vi "FTW-Container-Remove.vi"(0 "Container":refnum<class "FTW-Container.lvclass">, 5 "Value":variant, 11 "error in":errorcluster) -> (4 "Container out":refnum<class "FTW-Container.lvclass">, 6 "Removed?":bool, 8 "Value Removed":variant, 15 "error out":errorcluster)   [LabVIEW 2013, in "FTW-Container.lvclass"]
uses:
  FTW-Container.lvclass
panel:
  # "Inputs"
  # "Outputs"
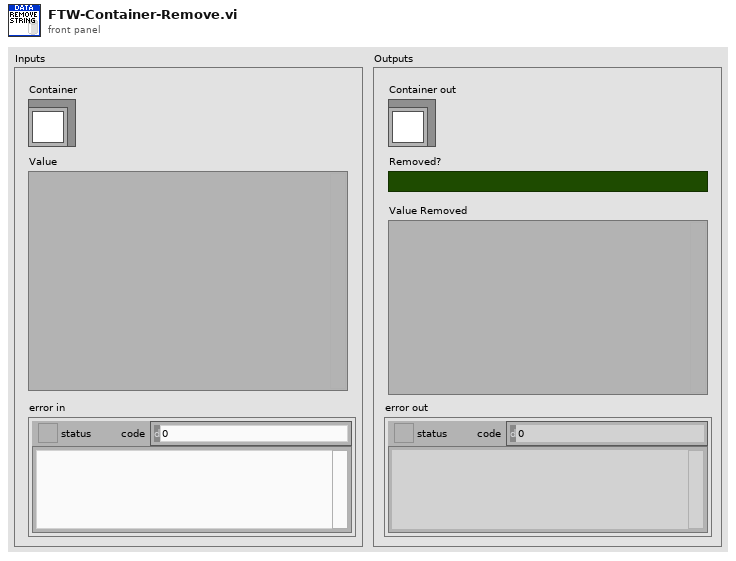
[diagram p1: front panel]
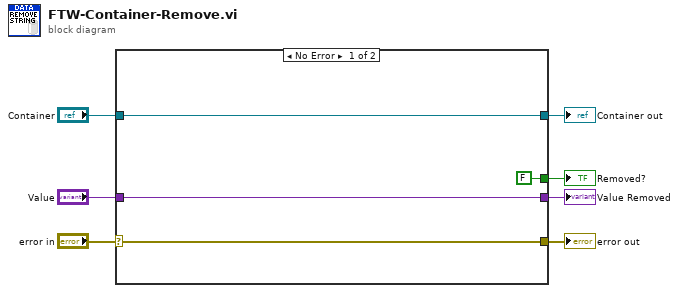
[diagram p0: block diagram]
diagram:
  n1 = case shown="No Error" "error in" {
    selector: "error in" -> [w9 w14]
    tunnel: [w9 w14] -> w7
    tunnel: [FALSE ("found") _] -> w5
    tunnel: "Container" -> [w11 w13]
    tunnel: [w11 w13] -> w3
    tunnel: "Value" -> [w10 w12]
    tunnel: [w10 w12] -> w2
    frame No Error {
    }
    frame Error {
    }
  }
  "error out" <- w7
  "Removed?" <- w5
  "Container out" <- w3
  "Value Removed" <- w2
